vi "Configure Connection Dialog - Resource Field.vi"(8 "error in (no error)":errorcluster, 9 "Current Connection":T2, 10 "Aliases":T3[](array[typedef]), 11 "Possible Connections":T6(array[cluster])=[{"Resource"="", "Possible Connections"=[]}, {"Resource"="", "Possible Connections"=[]}]) -> (0 "error out":errorcluster, 1 "Connection (R,S,D)":T1, 2 "Canceled?":bool, 3 "Connection":T2)   [LabVIEW 2017, in "Routing and Faulting System Explorer.lvlib"]
uses:
  Routing and Faulting System Explorer.lvlib
  Shared/Routing and Faulting Hardware API/Types/Possible Connections for Endpoint.ctl
  Connection Row.ctl
  Alias.ctl
  Endpoint.ctl
  Shared/Connection.ctl
  <vilib>/event_ctls.llb/lveventtype.ctl
  Shared/Routing and Faulting Hardware API/Routing and Faulting Hardware API.lvlib
  Shared/Routing and Faulting Shared.lvlib
panel:
  in  "Resource":string(combo)
  in  "Selected Source":string(combo)
  in  "Cancel Button":bool
  in  "OK Button":bool
  in  "Destination":string(combo)
  in  "Source":string(combo)
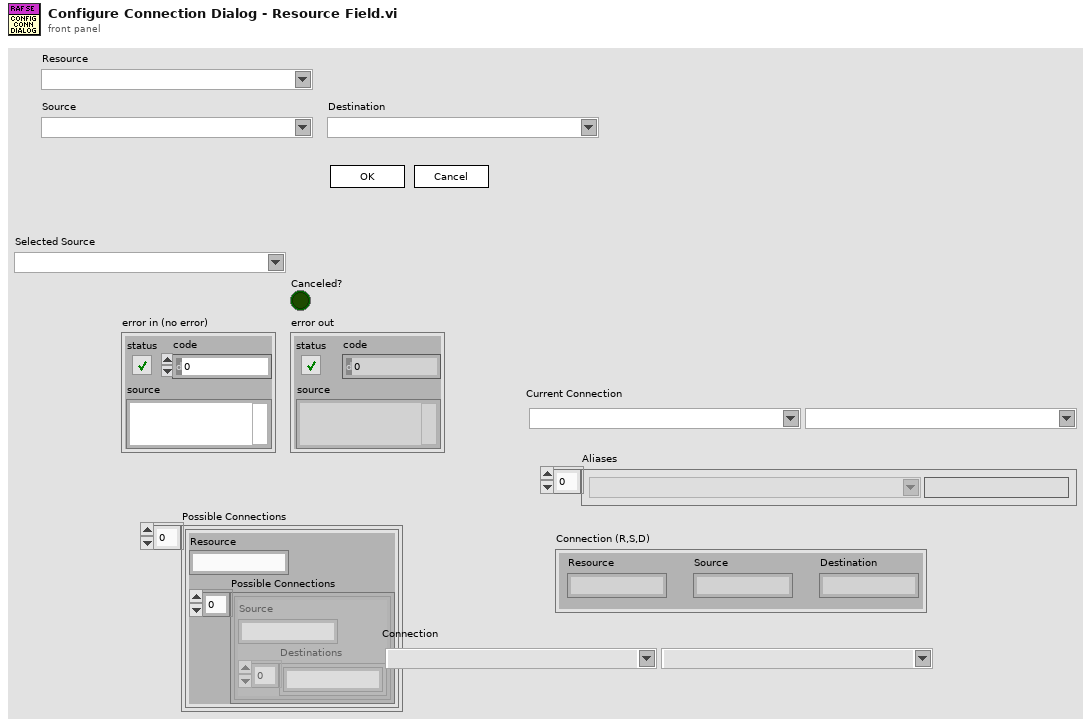
[diagram p1: front panel]
types:
  T1 = typedef "Routing and Faulting Shared.lvlib/Connection.ctl" = cluster{"Resource":string, "Source":string, "Destination":string}
  T2 = typedef "Routing and Faulting System Explorer.lvlib/Connection Row.ctl" = cluster{"Source":string, "Destination":string}
  T3 = typedef "Routing and Faulting System Explorer.lvlib/Alias.ctl" = cluster{"Endpoint":T4, "Alias":string}
  T4 = typedef "Routing and Faulting System Explorer.lvlib/Endpoint.ctl" = string
  T5 = typedef "Routing and Faulting Hardware API.lvlib/Possible Connections for Endpoint.ctl" = cluster{"Source":string, "Destinations":string[]}
  T6 = cluster{"Resource":string, "Possible Connections":T5[]}[]
  T7 = typedef "lveventtype.ctl" = enum32{"Null", "Timeout", "Annotation Menu Selection", "Annotation Menu Selection?", "App Instance Close", "App Instance Close?", "Autoscale Range Change", "Bookmark Info Change", "Cell Edit", "Cell Edit?", "Cursor Grab", "Cursor Grab?", "Cursor Menu Selection", "Cursor Menu Selection?", "Cursor Move", "Cursor Release", "Data Change", "Direction Change", "Display State Change", "Drag Ended", "Drag Enter", "Drag Leave", "Drag Over", "Drag Source Update", "Drag Starting", "Drag Starting?", "Drop", "Exec State Change", "Key Down", "Key Down?", "Key Repeat", "Key Repeat?", "Key Up", "Listbox Double Click", "Menu Activation?", "Menu Selection (App)", "Menu Selection? (App)", "Menu Selection (User)", "Mouse Down", "Mouse Down?", "Mouse Enter", "Mouse Leave", "Mouse Move", "Mouse Up", "Mouse Wheel", "NI Security User Change (App)", "Pane Size", "Panel Close", "Panel Close?", "Panel Resize", "Plot Attribute Change", "Scale Range Change", "Shortcut Menu Activation?", "Shortcut Menu Selection (App)", "Shortcut Menu Selection? (App)", "Shortcut Menu Selection (User)", "Tree Double Click", "Tree Drag", "Tree Drag?", "Tree Drop", "Tree Drop?", "Tree Item Close", "Tree Item Close?", "Tree Item Open", "Tree Item Open?", "User Event", "Value Change"}
  T8 = cluster{"Resource":string, "Possible Connections":T5[]}
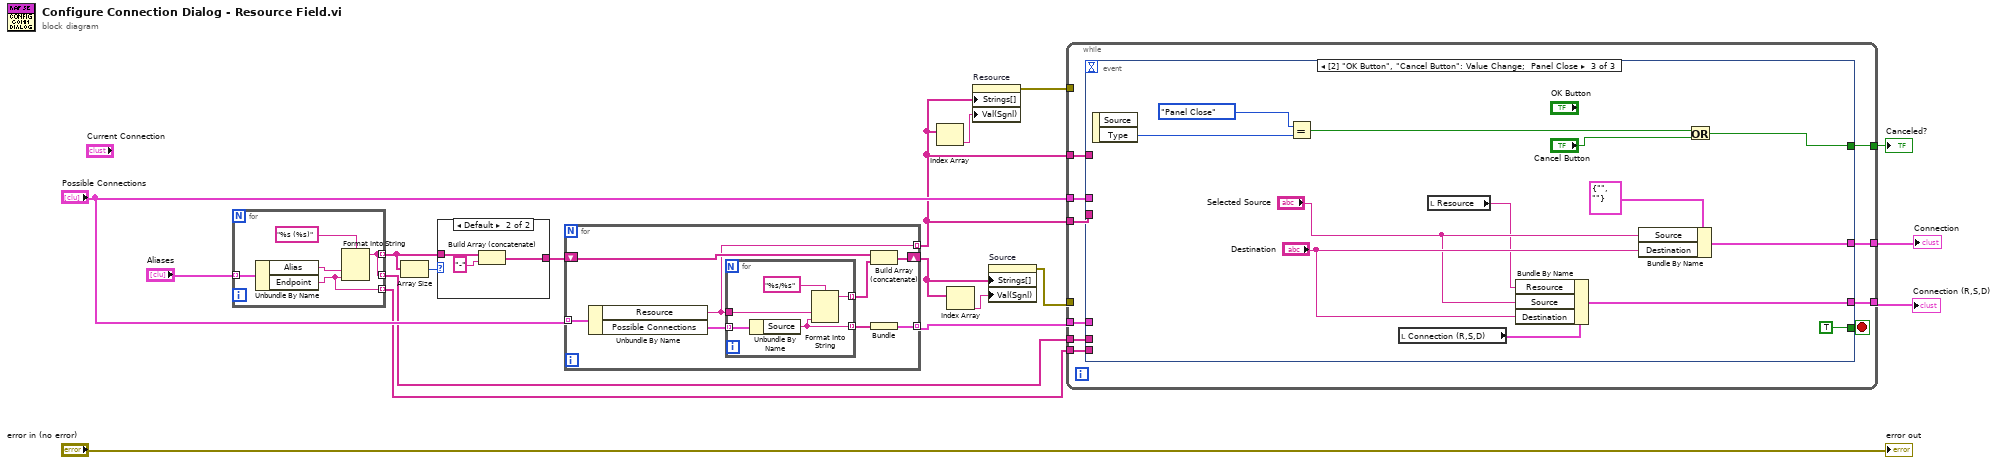
[diagram p0: block diagram]
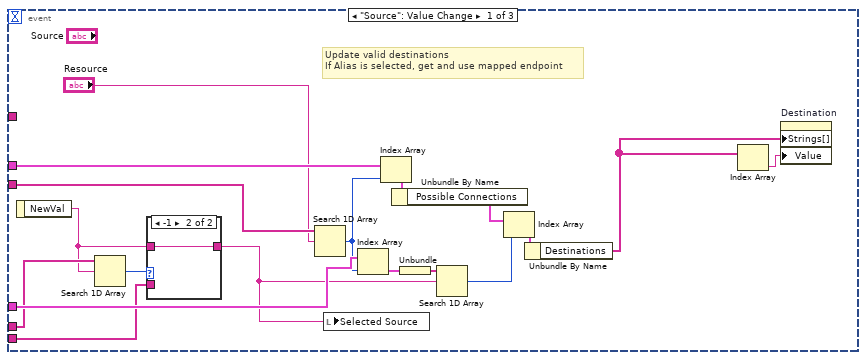
[diagram p3: hidden frame]
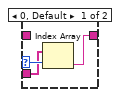
[diagram p4: hidden frame]
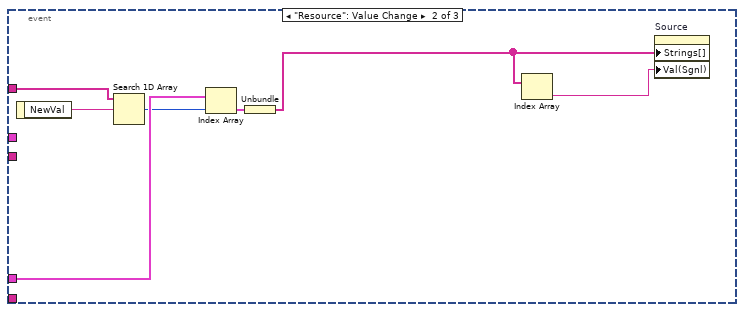
[diagram p5: hidden frame]
diagram:
  n1 = for {
    tunnel: "Aliases" -> [w23] mode=indexing
    tunnel: [w19] -> w13 mode=indexing
    tunnel: [w20] -> w5 mode=indexing
    tunnel: [w19] -> w4 mode=indexing
    n2 = Unbundle By Name(w23) -> ("Alias"=w21:string, "Endpoint"=w20:T4)
    n3 = Format Into String(format string="%s (%s)", w21, w20) -> (resulting string=w19:string)  [unwired: 2 in, 1 out]
  }
  n4 = Array Size(array=w13) -> (size(s)=w12:i32)
  n5 = case shown="Default" w12 {
    tunnel: w13 -> [w24 w27]
    tunnel: [w24 w25] -> w14
    frame 0 {
      # "No aliases.\nDon't add\nseparator"
    }
    frame Default {
      n6 = Build Array (concatenate)(w27, "-") -> (w25:string[])
    }
  }
  n7 = for {
    tunnel: "Possible Connections" -> [w35] mode=indexing
    shift-right: [w32] -> w8
    shift-left: w14 -> [w34]
    tunnel: [w31] -> w1 mode=indexing
    tunnel: [w28] -> w11 mode=indexing
    n8 = Unbundle By Name(w35) -> ("Resource"=w31:string, "Possible Connections"=w30:T5[])
    n9 = for {
      tunnel: w31 -> [w39]
      tunnel: [w38] -> w33 mode=indexing
      tunnel: w30 -> [w37] mode=indexing
      tunnel: [w36] -> w29 mode=indexing
      n10 = Unbundle By Name(w37) -> ("Source"=w36:string)
      n11 = Format Into String(format string="%s/%s", w39, w36) -> (resulting string=w38:string)  [unwired: 2 in, 1 out]
    }
    n12 = Build Array (concatenate)(w34, w33) -> (w32:string[])
    n13 = Bundle(w29) -> (w28:cluster{string[]})  [unwired: 1 in]
  }
  n14 = Index Array(array=w1) -> (element=w3:string)  [unwired: 1 in]
  n15 = Index Array(array=w8) -> (element=w9:string)  [unwired: 1 in]
  n16 = property on="Resource" class="CmbBox"("Strings[]"=w1, "Val(Sgnl)"=w3) -> (error out=w2:errorcluster)  [unwired: 2 in, 1 out]
  n17 = property on="Source" class="CmbBox"("Strings[]"=w8, "Val(Sgnl)"=w9) -> (error out=w6:errorcluster)  [unwired: 2 in, 1 out]
  n18 = while {
    tunnel: [w49] -> w18
    tunnel: "Possible Connections" -> [w48]
    tunnel: [w47] -> w16
    tunnel: w1 -> [w46]
    tunnel: w11 -> [w45]
    tunnel: [w44] -> w7
    tunnel: w6 -> [_]
    tunnel: w5 -> [w43]
    tunnel: w4 -> [w42]
    tunnel: w2 -> [_]
    tunnel: w1 -> [w41]
    stop <- w50 stop-if-true
    n19 = event shown="[2] \"OK Button\", \"Cancel Button\": Value Change;  Panel Close" {
      selector: _ -> [_ _ _]
      dyn-events: _ -> [_ _ _]
      timeout: _ -> [_ _ _]
      tunnel: [_ _ TRUE] -> w50
      tunnel: [_ _ w85] -> w49
      tunnel: w48 -> [w68 _ _]
      tunnel: [_ _ w90] -> w47
      tunnel: w46 -> [w55 _ _]
      tunnel: w45 -> [w66 w77 _]
      tunnel: [_ _ w83] -> w44
      tunnel: w43 -> [w53 _ _]
      tunnel: w42 -> [w57 _ _]
      tunnel: w41 -> [_ w79 _]
      event "Source": Value Change {
        # "Update valid destinations\nIf Alias is selected, get and use mapped endpoint"
        n20 = event-data() -> ("NewVal"=w54:string)  [unwired: 1 in]
        n21 = Search 1D Array(1D array=w57, element=w54) -> (index of element=w56:i32)  [unwired: 1 in]
        n22 = case shown="-1" w56 {
          selector: w56 -> [w71 _]
          tunnel: w54 -> [_ w72]
          tunnel: [w69 w72] -> w51
          tunnel: w53 -> [w70 _]
          frame 0, Default {
            n23 = Index Array(array=w70, index=w71) -> (element=w69:T4)
          }
          frame -1 {
          }
        }
        n24 = Search 1D Array(1D array=w55, element="Resource") -> (index of element=w65:i32)  [unwired: 1 in]
        n25 = local write "Selected Source"(w51) -> ()
        n26 = Index Array(array=w66, index=w65) -> (element=w64:cluster{string[]})
        n27 = Index Array(array=w68, index=w65) -> (element=w67:T8)
        n28 = Unbundle By Name(w67) -> ("Possible Connections"=w62:T5[])
        n29 = Unbundle(w64) -> (w63:string[])
        n30 = Search 1D Array(1D array=w63, element=w51) -> (index of element=w61:i32)  [unwired: 1 in]
        n31 = Index Array(array=w62, index=w61) -> (element=w60:T5)
        n32 = Unbundle By Name(w60) -> ("Destinations"=w58:string[])
        n33 = Index Array(array=w58) -> (element=w59:string)  [unwired: 1 in]
        n34 = property on="Destination" class="CmbBox"("Strings[]"=w58, "Value"=w59) -> ()  [unwired: 2 in, 2 out]
      }
      event "Resource": Value Change {
        n35 = event-data() -> ("NewVal"=w78:string)  [unwired: 1 in]
        n36 = Search 1D Array(1D array=w79, element=w78) -> (index of element=w76:i32)  [unwired: 1 in]
        n37 = Index Array(array=w77, index=w76) -> (element=w75:cluster{string[]})
        n38 = Unbundle(w75) -> (w74:string[])
        n39 = Index Array(array=w74) -> (element=w73:string)  [unwired: 1 in]
        n40 = property on="Source" class="CmbBox"("Strings[]"=w74, "Val(Sgnl)"=w73) -> ()  [unwired: 2 in, 2 out]
      }
      event "OK Button", "Cancel Button": Value Change; Panel Close {
        n41 = event-data() -> ("Type"=w88:T7)  [unwired: 1 in, 1 out]
        n42 = Equal?(x=lveventtype."Panel Close" ("Type"), y=w88) -> (x = y?=w87:bool)
        n43 = local read "Connection (R,S,D)"() -> (w84:T1)
        n44 = local read "Resource"() -> (w80:string)
        n45 = Bundle By Name(cluster=w84, "Resource"=w80, "Source"="Selected Source", "Destination"="Destination") -> (w83:T1)
        n46 = Bundle By Name(cluster=T2 {"Source"="", "Destination"=""} ("Connection"), "Source"="Selected Source", "Destination"="Destination") -> (w90:T2)
        n47 = Or(x=w87, y="Cancel Button") -> (x .or. y?=w85:bool)
      }
    }
  }
  "Canceled?" <- w18
  "Connection" <- w16
  "Connection (R,S,D)" <- w7
  "error out" <- "error in (no error)"
